vi "Execute.vi"(8 "error in (no error)":errorcluster, 11 "Scale in":refnum<class "Scale.lvclass">) -> (0 "error out":errorcluster, 2 "Data":dbl[](array[numeric]), 3 "Scale out":refnum<class "Scale.lvclass">)   [LabVIEW 2021, in "Scale.lvclass"]
uses:
  Scale.lvclass
  Scale.lvclass/Scale.ctl
  Decorator/Decorator.lvclass
  C:/PPLs/Decorator-Pattern/decorator-main/Presentation/Decorator/Decorator.lvclass
  C:/PPLs/Decorator-Pattern/decorator-main/Presentation/Component/Component.lvclass
  C:/PPLs/Decorator-Pattern/decorator-main/Presentation/Scale/Scale.lvclass
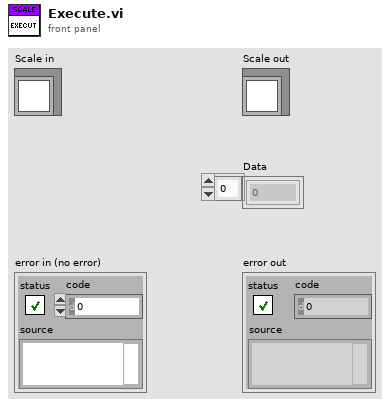
[diagram p1: front panel]
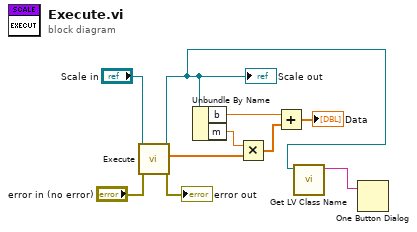
[diagram p0: block diagram]
diagram:
  n1 = call-parent "Execute.vi"("error in (no error)"="error in (no error)", "Decorator in"="Scale in") -> ("error out"=→"error out":errorcluster, "Data"=w6:dbl[], "Decorator out"=w1:refnum<class "Scale.lvclass">)  [unwired: 7 in]
  "Scale out" <- w1
  n2 = Unbundle By Name(w1) -> ("b"=w3:dbl, "m"=w5:dbl)
  n3 = Multiply(x=w5, y=w6) -> (x*y=w4:dbl[])
  n4 = Add(x=w3, y=w4) -> (x+y=→"Data":dbl[])
  n5 = call <vilib>:"Get LV Class Name.vi"("object"=w1) -> ("class name"=w2:string)  [unwired: 9 in, 1 out]
  n6 = One Button Dialog(message=w2) -> ()  [unwired: 1 in, 1 out]
